vi "Tipos de Datos.vi"() -> ()   [LabVIEW 2020]
panel:
  in  "Variant 2":variant
  out "Variant":variant
  out "Cluster 2":T1 {"Array 4" scale=0.0..100.0; "Meter" scale=0.0..10.0; "Knob" scale=0.0..10.0}
  in  "Cluster":T1 {"Array 4" scale=0.0..100.0; "Meter" scale=0.0..10.0; "Knob" scale=0.0..10.0}
  in  "Array 3":string[](array[string])
  out "Array 2":bool[](array[boolean])
  in  "Array":dbl[](array[slide]) scale=0.0..100.0
  out "String 2":string
  in  "String":string
  in  "Boolean 2":bool
  out "Boolean":bool
  out "Tank":u16(slide) scale=0.0..10.0
  in  "Slide":u16(slide) scale=0.0..10.0
  out "Meter":dbl(knob) scale=0.0..10.0
  in  "Thermometer":dbl(slide) scale=0.0..100.0
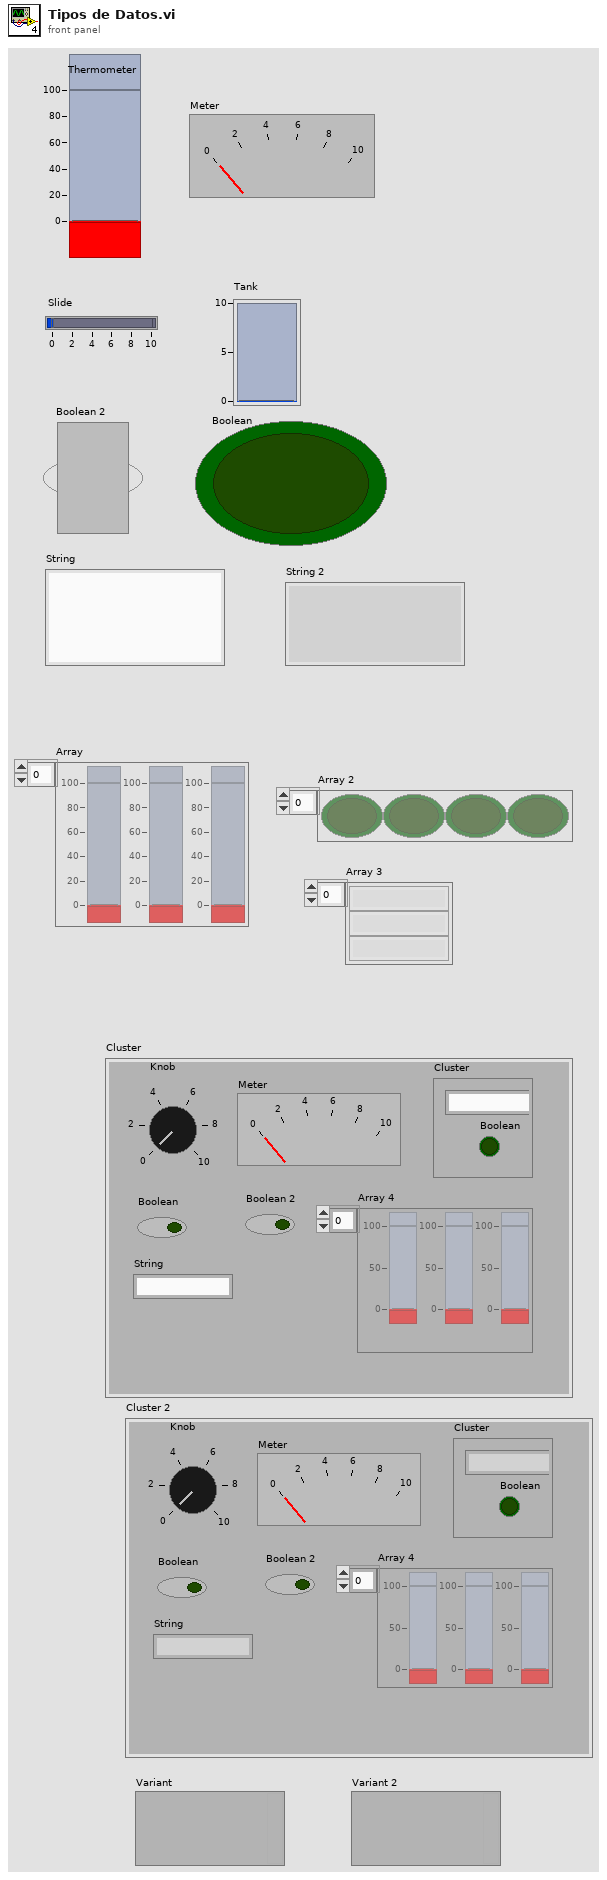
[diagram p1: front panel]
types:
  T1 = cluster{"Knob":dbl, "Meter":dbl, "Boolean":bool, "Boolean 2":bool, "String":string, "Array 4":dbl[], "Cluster":cluster{"String":string, "Boolean":bool}}
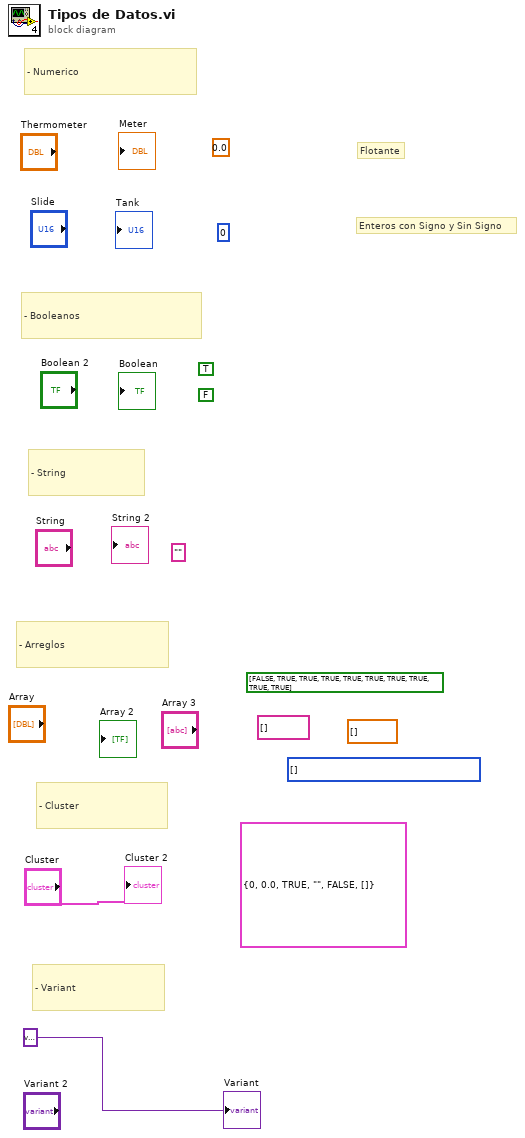
[diagram p0: block diagram]
diagram:
  (unwired) cluster{i32, dbl, bool, string, bool, dbl[]} {0, 0.0, TRUE, "", FALSE, []}
  (unwired) dbl[] []
  (unwired) string[] []
  (unwired) bool[] [FALSE, TRUE, TRUE, TRUE, TRUE, TRUE, TRUE, TRUE, TRUE, TRUE]
  (unwired) i32[] []
  (unwired) ""
  (unwired) FALSE
  (unwired) TRUE
  (unwired) 0
  (unwired) 0.0 ("Meter")
  # "Enteros con Signo y Sin Signo"
  # "Flotante"
  # "- Variant"
  # "- Arreglos"
  # "- Booleanos"
  # "- Cluster"
  # "- String"
  # "- Numerico"
  "Cluster 2" <- "Cluster"
  "Variant" <- variant
